vi "GUI LabVIEW Host PC.vi"() -> ()   [LabVIEW 2014]
doc: "The Serial - Monitoring GUI example shows best practices for a remote monitoring system with two VIs, one running on a host PC and the other running embedded in the Arduino compatible target. The example includes two-way serial communication between the host PC VI and the Arduino compatible target VI. This is the host PC VI which monitors and charts the sine wave data points that are generated and sent to the serial port by the embedded Arduino target VI. The host PC VI also includes the ability to pause and resume the sending of data points by the Arduino compatible target VI.\n\nFront Panel control parameters for each of the supported boards:\n\nUNO:\nArchitecture: avr\nBoard: uno\nCPU: left blank\n\nDUE:\nArchitecture: sam\nBoard: arduino_due_x_dbg (if USB cable connected to the debugging port) or arduino_due_x (if USB cable connected to the USB port)\nCPU: left blank\n\nNANO:\nArchitecture: avr\nBoard: nano\nCPU: atmega328 (if nano 3.x) or atmega168 (if nano 2.x)\n\nMEGA:\nArchitecture: avr\nBoard: megaADK\nCPU: left blank\n\nLEONARDO:\nArchitecture: avr\nBoard: leonardo\nCPU: left blank\n\nYUN:\nArchitecture: avr\nBoard: yun\nCPU: left blank"
uses:
  <vilib>/Instr/_visa.llb/VISA Configure Serial Port (Instr).vi
panel:
  out "Display 2":string="-"
  out "Display":string="-"
  in  "ESP8266 COM Port":string="COM6"
  in  "Stop":bool
  in  "Pause":bool
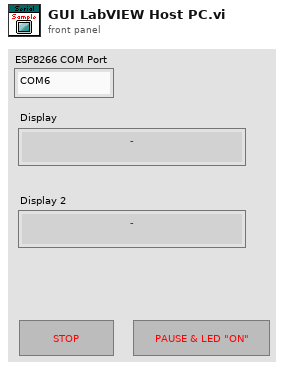
[diagram p1: front panel]
types:
  T1 = cluster{"baud rate":u32, "data bits":u16, "parity":enum16{"None", "Odd", "Even", "Mark", "Space"}, "stop bits":u16, "flow control":u16}
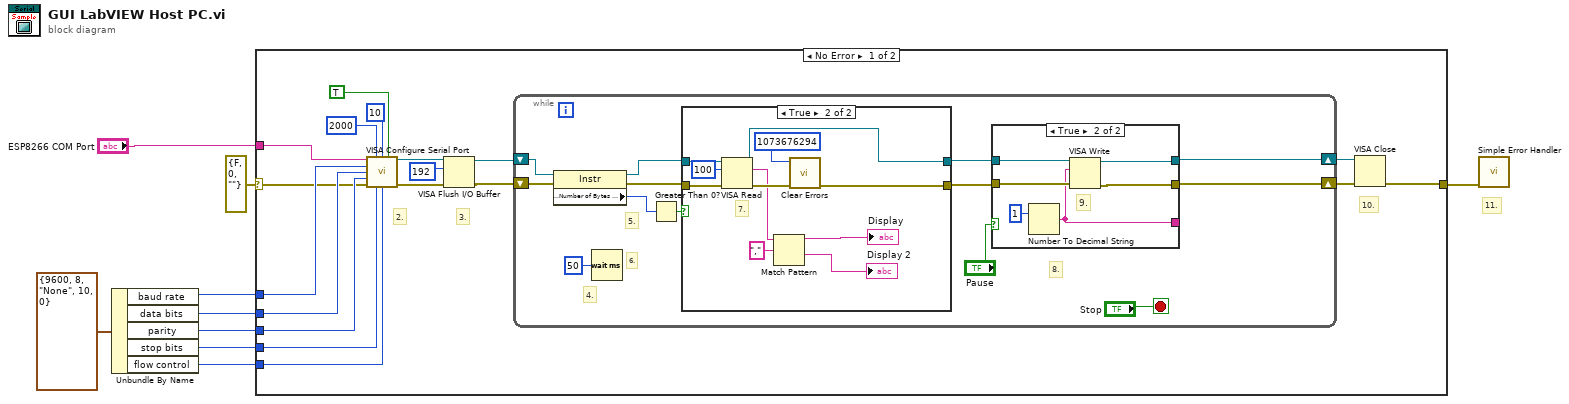
[diagram p0: block diagram]
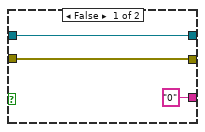
[diagram p2: hidden frame]
diagram:
  # "11."
  n1 = Unbundle By Name(T1 {"baud rate"=9600, "data bits"=8, "parity"=enum."None", "stop bits"=10, "flow control"=0} ("Serial Settings")) -> ("baud rate"=w8:u32, "data bits"=w7:u16, "parity"=w6:enum16{"None", "Odd", "Even", "Mark", "Space"}, "stop bits"=w5:u16, "flow control"=w4:u16)
  n2 = case shown="No Error" errorcluster {"status"=FALSE, "code"=0, "source"=""} ("error IO") {
    selector: errorcluster {"status"=FALSE, "code"=0, "source"=""} ("error IO") -> [w20 w63]
    tunnel: w8 -> [w27 _]
    tunnel: w7 -> [w26 _]
    tunnel: w6 -> [w25 _]
    tunnel: w5 -> [w24 _]
    tunnel: w4 -> [w23 _]
    tunnel: [w16 w63] -> w2
    tunnel: "ESP8266 COM Port" -> [w17 _]
    frame No Error {
      # "10."
      # "3."
      # "2."
      n3 = call-poly "VISA Configure Serial Port"("VISA resource name"=w17, "timeout (10sec)"=u32 2000, "termination char\n(0xA = '\\n' = LF)"=u8 10 ("termination char\n(0xA = '\\n' = LF)"), "Enable Termination\nChar (T)"=TRUE ("Enable Termination\nChar (T)"), "baud rate (9600)"=w27, "data bits (8)"=w26, "parity (0:none)"=w25, "error in (no error)"=w20, "stop bits (10: 1 bit)"=w24, "flow control (0:none)"=w23) -> ("VISA resource name out"=w18:refnum<visa-resource-name>, "error out"=w19:errorcluster)  [unwired: 4 out]
      n4 = VISA Flush I/O Buffer(VISA resource name=w18, mask (16)=u16 192, error in (no error)=w19) -> (VISA resource name out=w14:refnum<visa-resource-name>, error out=w13:errorcluster)
      n5 = while {
        shift-right: [w30] -> w11
        shift-left: w13 -> [w39]
        shift-right: [w28] -> w12
        shift-left: w14 -> [w38]
        stop <- "Stop" stop-if-true
        # "8."
        # "6."
        # "5."
        # "4."
        n6 = property class="Instr"(reference=w38, error in=w39) -> (reference out=w40:refnum<visa-resource-name>, error out=w37:errorcluster, "Serial Settings:Number of Bytes at Serial Port"=w36:u32)
        n7 = Wait (ms)(milliseconds to wait=u32 50) -> ()  [unwired: 1 out]
        n8 = Greater Than 0?(x=w36) -> (x > 0?=w35:bool)
        n9 = case shown="True" w35 {
          tunnel: [w51 w62] -> w32
          tunnel: w40 -> [w51 w61]
          tunnel: w37 -> [w50 w60]
          tunnel: [w50 w57] -> w31
          frame False {
          }
          frame True {
            # "7."
            n10 = VISA Read(VISA resource name=w61, byte count=u32 100, error in (no error)=w60) -> (VISA resource name out=w62:refnum<visa-resource-name>, read buffer=w55:string, error out=w59:errorcluster)  [unwired: 1 out]
            n11 = Match Pattern(string=w55, regular expression=",") -> (before substring=→"Display":string, after substring=→"Display 2":string)  [unwired: 1 in, 2 out]
            n12 = call <vilib>:"Clear Errors.vi"("error in (no error)"=w59, "specific error code to clear (0: all)"=1073676294) -> ("error out"=w57:errorcluster)  [unwired: 4 in, 1 out]
          }
        }
        n13 = case shown="True" "Pause" {
          tunnel: w32 -> [w42 w48]
          tunnel: w31 -> [w43 w47]
          tunnel: [w43 w46] -> w30
          tunnel: [w42 w45] -> w28
          tunnel: ["0" w44] -> _
          frame False {
          }
          frame True {
            # "9."
            n14 = Number To Decimal String(number=u32 1 ("milliseconds to wait")) -> (decimal integer string=w44:string)  [unwired: 1 in]
            n15 = VISA Write(VISA resource name=w48, write buffer=w44, error in (no error)=w47) -> (VISA resource name out=w45:refnum<visa-resource-name>, error out=w46:errorcluster)  [unwired: 1 out]
          }
        }
      }
      n16 = VISA Close(VISA resource name=w12, error in (no error)=w11) -> (error out=w16:errorcluster)
    }
    frame Error {
    }
  }
  n17 = call <vilib>:"Simple Error Handler.vi"("error in (no error)"=w2) -> ()  [unwired: 4 in, 5 out]
